vi "Agitate to Spin.vi"(0 "GEA2 Reference In":refnum<k24>, 1 "Standalone?":bool, 2 "Upper Limits":dbl[][](array[numeric])=[[0.0, 0.08, 4.1], [3.2, 0.08, 1.1]], 5 "GEA Inputs":T1 {"Destination" format="%.0x"; "Source" format="%.0x"}, 7 "Shift without testing?":bool, 11 "Error In":errorcluster, 13 "Lower Limits":dbl[][](array[numeric])=[[0.0, 0.02, 3.8], [2.9, 0.02, 0.7]]) -> (4 "GEA2 Reference Out":refnum<k24>, 6 "Pass/Fail?":bool, 8 "Report Text":string, 15 "Error Out":errorcluster)   [LabVIEW 2016, in "2015 VA Washer.lvlib"]
uses:
  Projects/2015 VA Washer.lvlib
  C:/Automation/DLLs/PC Dot Net/GeaCommunication.dll
  Common/LabVIEW GEA2 Toolkit/LabVIEW_GEA2_Toolkit.lvlibp/type defs/Source_Destination.ctl
  Common/LabVIEW GEA2 Toolkit/LabVIEW_GEA2_Toolkit.lvlibp/type defs/ERD Write Data In.ctl
  Common/LabVIEW GEA2 Toolkit/LabVIEW_GEA2_Toolkit.lvlibp/type defs/Data Type.ctl
  Common/LabVIEW GEA2 Toolkit/LabVIEW_GEA2_Toolkit.lvlibp/type defs/ERD Read Data In.ctl
  Valew Common/type defs/MC_Cycle_Engine_Request_State.ctl
  <vilib>/DAQmx/write.llb/DAQmx Write (Digital Bool 1Line 1Point).vi
  <vilib>/DAQmx/create/channels.llb/DAQmx Create Channel (DO-Digital Output).vi
  <vilib>/DAQmx/miscellaneous.llb/DAQmx Fill In Error Info.vi
  Common/LabVIEW GEA2 Toolkit/LabVIEW_GEA2_Toolkit.lvlibp
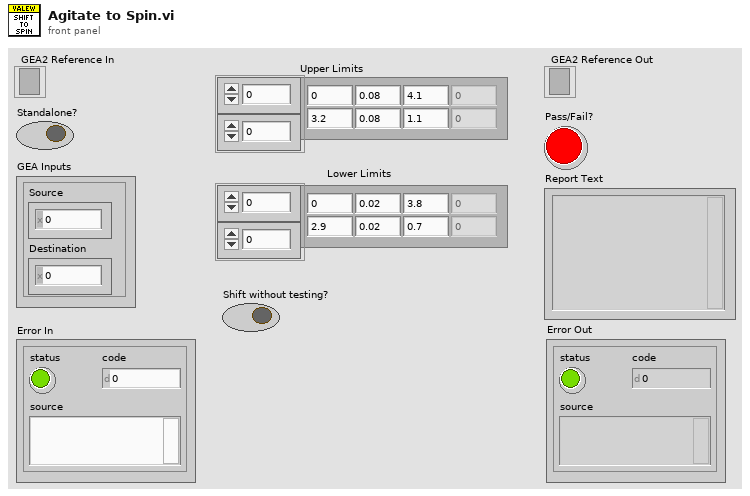
[diagram p1: front panel]
types:
  T1 = typedef "LabVIEW_GEA2_Toolkit.lvlibp/Source_Destination.ctl" = cluster{"Source":u8, "Destination":u8}
  T2 = enum16{"EQ (==)", "NE (!=)", "GT (>)", "LT (<)", "GE (>=)", "LE (<=)", "GTLT(> <)", "GELE (>= <=)", "GELT (>= <)", "GTLE (> <=)", "LTGT (< >)", "LEGE (<= >=)", "LEGT (<= >)", "LTGE (< >=)", "No Comparison"}
  T3 = typedef "LabVIEW_GEA2_Toolkit.lvlibp/ERD Read Data In.ctl" = cluster{"ERD Number":u16, "Data Type":T4}
  T4 = typedef "LabVIEW_GEA2_Toolkit.lvlibp/Data Type.ctl" = enum16{"string", "boolean", "uint8_t", "uint16_t", "uint32_t", "uint64_t", "int8_t", "int16_t", "int32_t", "int64_t"}
  T5 = typedef "LabVIEW_GEA2_Toolkit.lvlibp/ERD Write Data In.ctl" = cluster{"ERD Number":u16, "Data Type":T4, "Data":string}
  T6 = typedef "LabVIEW_GEA2_Toolkit.lvlibp/ERD Read Data Out.ctl" = cluster{"ERD Number":u16, "Data":string}
  T7 = typedef "2015 VA Washer.lvlib/MC_Cycle_Engine_Request_State.ctl" = enum16{"Select", "Start", "Pause", "Resume", "Stop"}
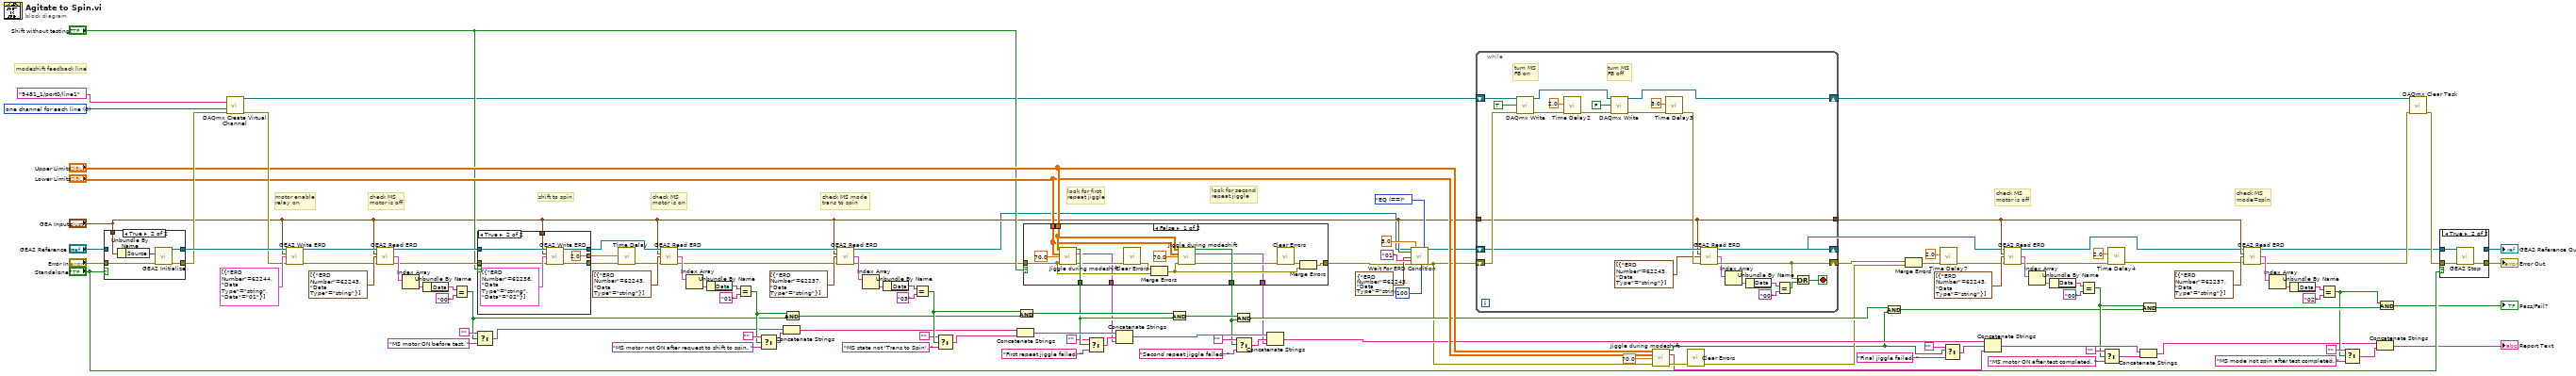
[diagram p0: block diagram]
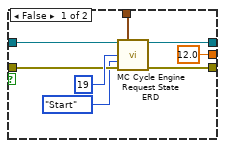
[diagram p2: hidden frame]
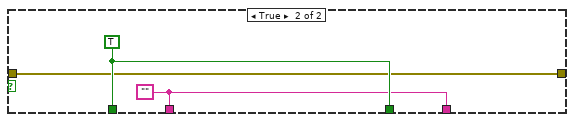
[diagram p3: hidden frame]
diagram:
  w126 = 0 items=["one channel for each line", "one channel for all lines"] ("line grouping")
  # "modeshift feedback line"
  # "look for second\nrepeat jiggle"
  # "look for first\nrepeat jiggle"
  # "check MS\nmode=spin"
  # "check MS\nmotor is off"
  # "check MS mode\ntrans to spin"
  # "check MS\nmotor is on"
  # "shift to spin"
  # "check MS\nmotor is off"
  # "motor enable\nrelay on"
  n1 = case shown="True" "Standalone?" {
    tunnel: [w128 w134] -> w118
    tunnel: "Error In" -> [w129 w130]
    tunnel: [w129 w133] -> w77
    tunnel: "GEA2 Reference In" -> [w128 _]
    tunnel: "GEA Inputs" -> [_ w132]
    frame False {
    }
    frame True {
      n2 = Unbundle By Name(w132) -> ("Source"=w131:u8)
      n3 = call "GEA2 Initialize.vi"("Source Address"=w131, "error in"=w130) -> ("GEA2 Reference Out"=w134:refnum<k24>, "error out"=w133:errorcluster)  [unwired: 11 in, 1 out]
    }
  }
  n4 = call-poly <vilib>:"DAQmx Create Virtual Channel.vi"("lines"=tag "9481_1/port0/line1", "line grouping"=w126, "error in"=w77) -> ("task out"=w20:refnum<k21>, "error out"=w76:errorcluster)  [unwired: 11 in]
  n5 = call "GEA2 Write ERD.vi"("GEA2 Reference In"=w118, "GEA Inputs"="GEA Inputs", "Write ERD List"=T5[] [{"ERD Number"=62244, "Data Type"=enum."string", "Data"="01"}], "Error In"=w76) -> ("GEA2 Reference Out"=w117:refnum<k24>, "Error Out"=w116:errorcluster)  [unwired: 9 in, 1 out]
  n6 = call "GEA2 Read ERD.vi"("GEA2 Reference In"=w117, "GEA Inputs"="GEA Inputs", "Read ERD List"=T3[] [{"ERD Number"=62243, "Data Type"=enum."string"}], "Error In"=w116) -> ("GEA2 Reference Out"=w110:refnum<k24>, "ERD Data Out"=w122:T6[], "Error Out"=w109:errorcluster)  [unwired: 8 in, 1 out]
  n7 = Index Array(array=w122) -> (element=w121:T6)  [unwired: 1 in]
  n8 = Unbundle By Name(w121) -> ("Data"=w119:string)
  n9 = Equal?(x=w119, y="00") -> (x = y?=w99:bool)
  n10 = Select(t="", s=w99, f="MS motor ON before test. " ("y")) -> (s? t:f=w98:string)
  n11 = case shown="True" "Shift without testing?" {
    tunnel: w110 -> [w140 w148]
    tunnel: w109 -> [w141 w147]
    tunnel: [w138 w146] -> w101
    tunnel: [w137 w145] -> w84
    tunnel: "GEA Inputs" -> [w139 w144]
    tunnel: [12.0 ("Delay Time (s)") 2.0 ("Delay Time (s)")] -> w32
    frame False {
      n12 = call "MC Cycle Engine Request State ERD.vi"("GEA2 Reference In"=w140, "GEA Inputs"=w139, "Cycle #"=u8 19, "MC Cycle Engine State"=MC_Cycle_Engine_Request_State."Start", "Error In"=w141) -> ("GEA2 Reference Out"=w138:refnum<k24>, "Error Out"=w137:errorcluster)  [unwired: 9 in]
    }
    frame True {
      n13 = call "GEA2 Write ERD.vi"("GEA2 Reference In"=w148, "GEA Inputs"=w144, "Write ERD List"=T5[] [{"ERD Number"=62238, "Data Type"=enum."string", "Data"="02"}], "Error In"=w147) -> ("GEA2 Reference Out"=w146:refnum<k24>, "Error Out"=w145:errorcluster)  [unwired: 9 in, 1 out]
    }
  }
  n14 = call "Time Delay"("error in (no error)"=w84, "Delay Time (s)"=w32) -> ("error out"=w83:errorcluster)  [unwired: 9 in]
  n15 = call "GEA2 Read ERD.vi"("GEA2 Reference In"=w101, "GEA Inputs"="GEA Inputs", "Read ERD List"=T3[] [{"ERD Number"=62243, "Data Type"=enum."string"}], "Error In"=w83) -> ("GEA2 Reference Out"=w87:refnum<k24>, "ERD Data Out"=w108:T6[], "Error Out"=w85:errorcluster)  [unwired: 8 in, 1 out]
  n16 = Index Array(array=w108) -> (element=w107:T6)  [unwired: 1 in]
  n17 = Unbundle By Name(w107) -> ("Data"=w105:string)
  n18 = Equal?(x=w105, y="01") -> (x = y?=w100:bool)
  n19 = Select(t="", s=w100, f="MS motor not ON after request to shift to spin. " ("y")) -> (s? t:f=w97:string)
  n20 = Concatenate Strings(w98, w97) -> (w86:string)
  n21 = And(x=w100, y=w99) -> (x .and. y?=w82:bool)
  n22 = call "GEA2 Read ERD.vi"("GEA2 Reference In"=w87, "GEA Inputs"="GEA Inputs", "Read ERD List"=T3[] [{"ERD Number"=62237, "Data Type"=enum."string"}], "Error In"=w85) -> ("GEA2 Reference Out"=w21:refnum<k24>, "ERD Data Out"=w88:T6[], "Error Out"=w16:errorcluster)  [unwired: 8 in, 1 out]
  n23 = Index Array(array=w88) -> (element=w89:T6)  [unwired: 1 in]
  n24 = Unbundle By Name(w89) -> ("Data"=w91:string)
  n25 = Equal?(x=w91, y="03") -> (x = y?=w95:bool)
  n26 = Select(t="", s=w95, f="MS state not 'Trans to Spin'. " ("y")) -> (s? t:f=w96:string)
  n27 = Concatenate Strings(w86, w96) -> (w80:string)
  n28 = And(x=w95, y=w82) -> (x .and. y?=w81:bool)
  n29 = case shown="False" "Shift without testing?" {
    tunnel: w16 -> [w155 w166]
    tunnel: "Upper Limits" -> [w162 _]
    tunnel: "Lower Limits" -> [w161 _]
    tunnel: [w160 w167] -> w43
    tunnel: [w159 w167] -> w37
    tunnel: [w154 w166] -> w14
    tunnel: [w151 w165] -> w8
    tunnel: [w150 w165] -> w7
    frame False {
      n30 = call "Jiggle during modeshift.vi"("Upper Limits"=w162, "Lower Limits"=w161, "Timeout (s)"=70.0, "Error In"=w155) -> ("Pass/Fail?"=w160:bool, "Report Text"=w151:string, "Error Out"=w158:errorcluster)  [unwired: 8 in, 1 out]
      n31 = call <vilib>:"Clear Errors.vi"("error in (no error)"=w158) -> ("error out"=w156:errorcluster)  [unwired: 5 in, 1 out]
      n32 = Merge Errors(w156, w155) -> (w152:errorcluster)
      n33 = call "Jiggle during modeshift.vi"("Upper Limits"=w162, "Lower Limits"=w161, "Timeout (s)"=70.0, "Error In"=w152) -> ("Pass/Fail?"=w159:bool, "Report Text"=w150:string, "Error Out"=w157:errorcluster)  [unwired: 8 in, 1 out]
      n34 = call <vilib>:"Clear Errors.vi"("error in (no error)"=w157) -> ("error out"=w153:errorcluster)  [unwired: 5 in, 1 out]
      n35 = Merge Errors(w153, w152) -> (w154:errorcluster)
    }
    frame True {
      w165 = ""
      w167 = TRUE ("Pass/Fail?")
    }
  }
  n36 = Select(t="", s=w43, f="First repeat jiggle failed. " ("y")) -> (s? t:f=w44:string)
  n37 = Concatenate Strings(w80, w44, w8) -> (w78:string)
  n38 = And(x=w81, y=w43) -> (x .and. y?=w79:bool)
  n39 = And(x=w79, y=w37) -> (x .and. y?=w29:bool)
  n40 = Select(t="", s=w37, f="Second repeat jiggle failed. " ("y")) -> (s? t:f=w39:string)
  n41 = Concatenate Strings(w78, w39, w7) -> (w30:string)
  n42 = call "Wait For ERD Condition.vi"("GEA2 Reference In"=w21, "GEA Inputs"="GEA Inputs", "ERD Read Data"=T3 {"ERD Number"=62243, "Data Type"=enum."string"} ("ERD Read Data In"), "Expected Low"="01", "Error In"=w14, "Timeout (s)"=5.0, "Loop Rate (ms)"=u32 100, "Comparison"=T2."EQ (==)") -> ("GEA2 Reference Out"=w26:refnum<k24>, "Error Out"=w11:errorcluster)  [unwired: 7 in, 3 out]
  n43 = while {
    shift-right: [w172] -> w9
    shift-left: w11 -> [w175]
    shift-right: [w180] -> w17
    shift-left: w20 -> [w181]
    shift-right: [w168] -> w18
    shift-left: w26 -> [w174]
    tunnel: "GEA Inputs" -> [w171]
    tunnel: [w171] -> w19
    stop <- w177 stop-if-true
    # "turn MS\nFB on"
    # "turn MS\nFB off"
    n44 = call-poly <vilib>:"DAQmx Write.vi"("task/channels in"=w181, "data"=TRUE, "error in"=w175) -> ("task out"=w183:refnum<k21>, "error out"=w184:errorcluster)  [unwired: 10 in, 1 out]
    n45 = call "Time Delay2"("error in (no error)"=w184, "Delay Time (s)"=2.0) -> ("error out"=w182:errorcluster)  [unwired: 9 in]
    n46 = call-poly <vilib>:"DAQmx Write.vi"("task/channels in"=w183, "data"=FALSE, "error in"=w182) -> ("task out"=w180:refnum<k21>, "error out"=w178:errorcluster)  [unwired: 10 in, 1 out]
    n47 = call "Time Delay3"("error in (no error)"=w178, "Delay Time (s)"=3.0) -> ("error out"=w173:errorcluster)  [unwired: 9 in]
    n48 = call "GEA2 Read ERD.vi"("GEA2 Reference In"=w174, "GEA Inputs"=w171, "Read ERD List"=T3[] [{"ERD Number"=62243, "Data Type"=enum."string"}], "Error In"=w173) -> ("GEA2 Reference Out"=w168:refnum<k24>, "ERD Data Out"=w169:T6[], "Error Out"=w172:errorcluster)  [unwired: 8 in, 1 out]
    n49 = Index Array(array=w169) -> (element=w190:T6)  [unwired: 1 in]
    n50 = Unbundle By Name(w190) -> ("Data"=w189:string)
    n51 = Equal?(x=w189, y="00") -> (x = y?=w176:bool)
    n52 = Or(x=w172, y=w176) -> (x .or. y?=w177:bool)
  }
  n53 = call "Jiggle during modeshift.vi"("Upper Limits"="Upper Limits", "Lower Limits"="Lower Limits", "Timeout (s)"=70.0, "Error In"=w11) -> ("Pass/Fail?"=w6:bool, "Report Text"=w5:string, "Error Out"=w15:errorcluster)  [unwired: 8 in, 1 out]
  n54 = call <vilib>:"Clear Errors.vi"("error in (no error)"=w15) -> ("error out"=w10:errorcluster)  [unwired: 5 in, 1 out]
  n55 = And(x=w29, y=w6) -> (x .and. y?=w65:bool)
  n56 = Merge Errors(w9, w10) -> (w13:errorcluster)
  n57 = call "Time Delay7"("error in (no error)"=w13, "Delay Time (s)"=2.0) -> ("error out"=w45:errorcluster)  [unwired: 9 in]
  n58 = Select(t="", s=w6, f="Final jiggle failed. " ("y")) -> (s? t:f=w34:string)
  n59 = Concatenate Strings(w30, w34, w5) -> (w68:string)
  n60 = call "GEA2 Read ERD.vi"("GEA2 Reference In"=w18, "GEA Inputs"=w19, "Read ERD List"=T3[] [{"ERD Number"=62243, "Data Type"=enum."string"}], "Error In"=w45) -> ("GEA2 Reference Out"=w1:refnum<k24>, "ERD Data Out"=w75:T6[], "Error Out"=w4:errorcluster)  [unwired: 8 in, 1 out]
  n61 = Index Array(array=w75) -> (element=w74:T6)  [unwired: 1 in]
  n62 = Unbundle By Name(w74) -> ("Data"=w72:string)
  n63 = Equal?(x=w72, y="00") -> (x = y?=w66:bool)
  n64 = Select(t="", s=w66, f="MS motor ON after test completed. " ("y")) -> (s? t:f=w67:string)
  n65 = call "Time Delay4"("error in (no error)"=w4, "Delay Time (s)"=2.0) -> ("error out"=w3:errorcluster)  [unwired: 9 in]
  n66 = Concatenate Strings(w68, w67) -> (w55:string)
  n67 = And(x=w66, y=w65) -> (x .and. y?=w57:bool)
  n68 = call "GEA2 Read ERD.vi"("GEA2 Reference In"=w1, "GEA Inputs"=w19, "Read ERD List"=T3[] [{"ERD Number"=62237, "Data Type"=enum."string"}], "Error In"=w3) -> ("GEA2 Reference Out"=w51:refnum<k24>, "ERD Data Out"=w64:T6[], "Error Out"=w53:errorcluster)  [unwired: 8 in, 1 out]
  n69 = Index Array(array=w64) -> (element=w63:T6)  [unwired: 1 in]
  n70 = Unbundle By Name(w63) -> ("Data"=w61:string)
  n71 = Equal?(x=w61, y="02") -> (x = y?=w56:bool)
  n72 = Select(t="", s=w56, f="MS mode not spin after test completed. " ("y")) -> (s? t:f=w54:string)
  n73 = Concatenate Strings(w55, w54) -> (→"Report Text":string)
  n74 = And(x=w56, y=w57) -> (x .and. y?=→"Pass/Fail?":bool)
  n75 = call <vilib>:"DAQmx Clear Task.vi"("task in"=w17, "error in"=w53) -> ("error out"=w52:errorcluster)  [unwired: 13 in]
  n76 = case shown="True" "Standalone?" {
    tunnel: w51 -> [w192 w195]
    tunnel: w52 -> [w191 w194]
    tunnel: [w192 _] -> w123
    tunnel: [w191 w193] -> w12
    frame False {
    }
    frame True {
      n77 = call "GEA2 Stop.vi"("GEA2 Reference In"=w195, "Error In"=w194) -> ("Error Out"=w193:errorcluster)  [unwired: 13 in]
    }
  }
  "GEA2 Reference Out" <- w123
  "Error Out" <- w12
